vi "Final PID.vi"() -> ()   [LabVIEW 2009, in "Varian Magnet.lvclass"]
uses:
  Varian Magnet.lvclass
  <vilib>/DAQmx/create/channels.llb/DAQmx Create Channel (AO-Voltage-Basic).vi
  <vilib>/DAQmx/configure/timing.llb/DAQmx Timing (Sample Clock).vi
  <vilib>/DAQmx/create/channels.llb/DAQmx Create Channel (AI-Voltage-Basic).vi
  <vilib>/DAQmx/read.llb/DAQmx Read (Analog 1D DBL 1Chan NSamp).vi
  <vilib>/DAQmx/write.llb/DAQmx Write (Analog DBL 1Chan 1Samp).vi
  <vilib>/Analysis/NI_AALBase.lvlib
panel:
  in  "error in":errorcluster
  out "At Field":bool
  in  "stop 2":bool
  in  "Go to Field":bool
  in  "Field Desired (T)":dbl min=0.0 max=1.2 step=0.1
  out "Tesla":dbl(knob) scale=0.0..1.25
  out "Set Field":dbl min=0.0 max=1.25 step=0.001
  out "Magnetic Field":dbl(graph)
  in  "stop":bool
  in  "data":dbl min=-9.0 max=9.0 format="%0.2f"
  # "Big Knob Ranges:\n0  :  0 T\n10:   0T -.3 T \n20:   0T - .55T\n30:   0T - .8 T \n40:   0T - 1.02T \n50: .05T- 1.13T \n60: .25T- >1.13T \n70: .45T- >1.13T"
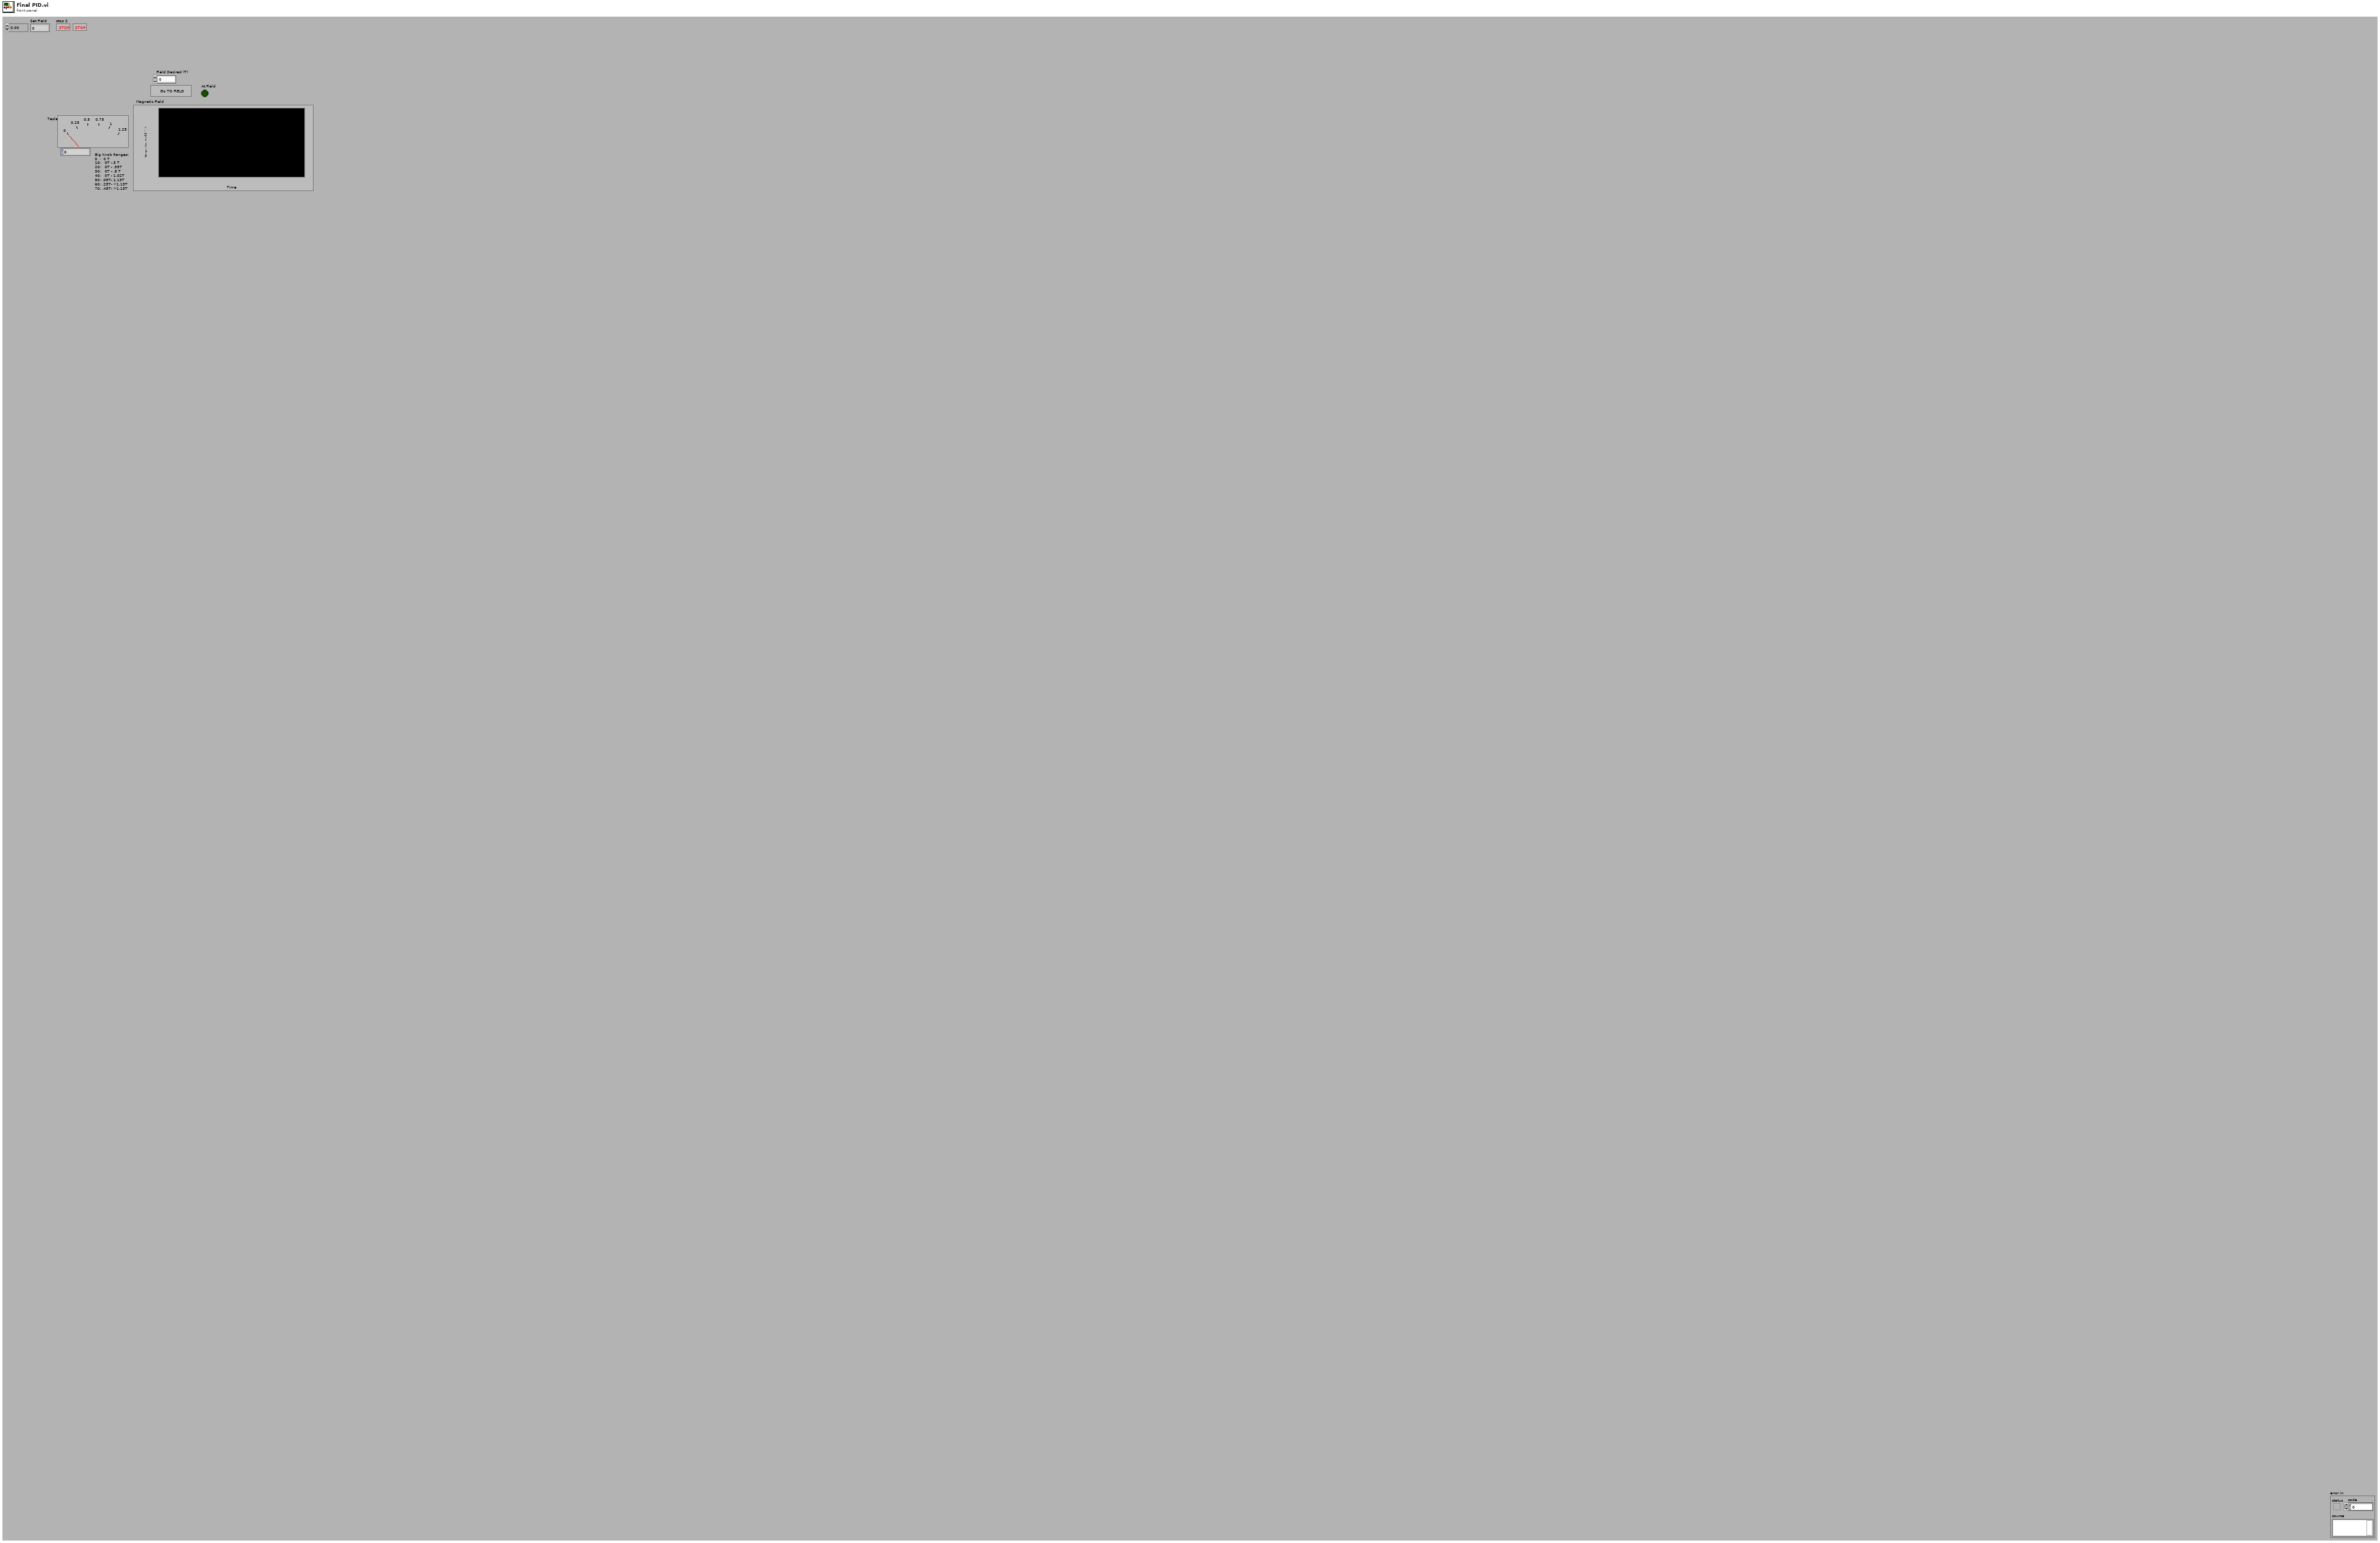
[diagram p1: front panel]
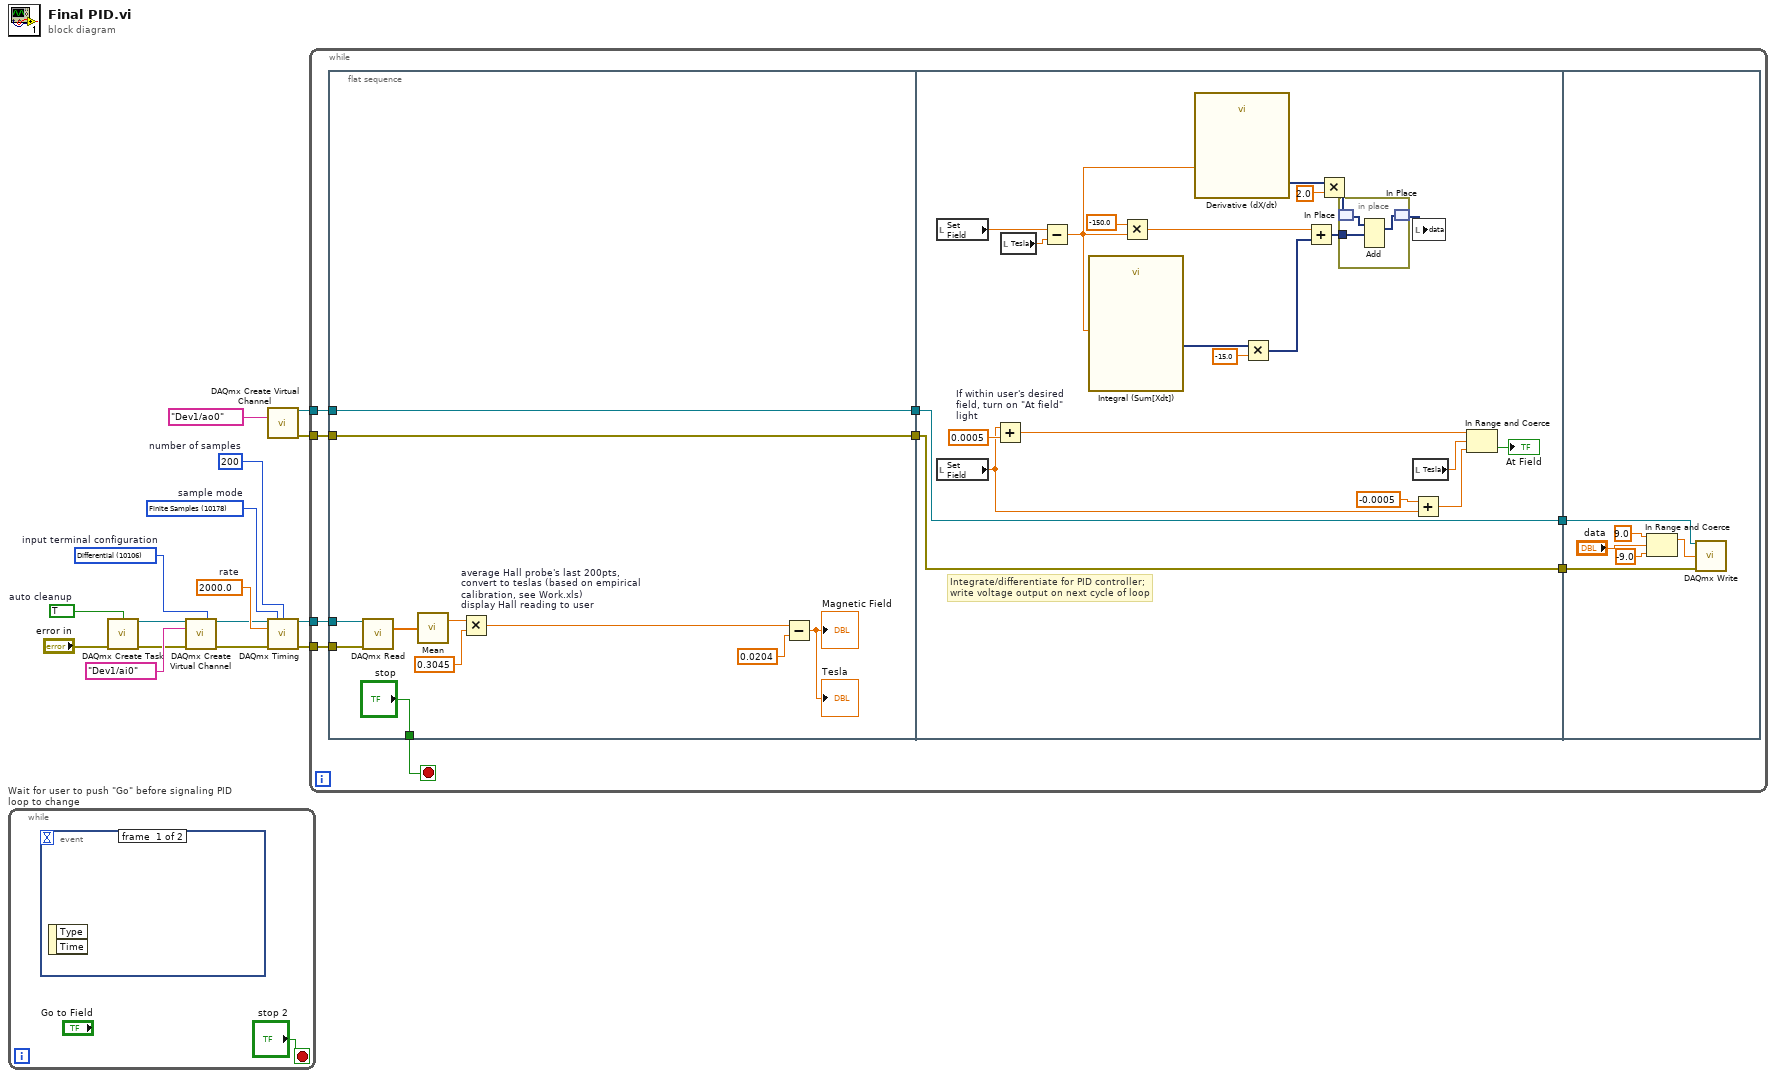
[diagram p0: block diagram]
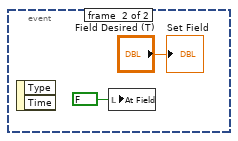
[diagram p2: hidden frame]
diagram:
  w13 = 10178 items=["Finite Samples"=10178, "Continuous Samples"=10123, "Hardware Timed Single Point"=12522]  # sample mode
  w12 = 200  # number of samples
  w11 = 2000.0  # rate
  w4 = 10106 items=["default"=-1, "RSE"=10083, "NRSE"=10078, "Differential"=10106, "Pseudodifferential"=12529]  # input terminal configuration
  w10 = TRUE  # auto cleanup
  n1 = while "Wait for user to push \"Go\" before signaling PID loop to change" {
    stop <- "stop 2" stop-if-true
    n2 = event shown="[1] \"Go to Field\": Value Change" {
      selector: _ -> [_ _]
      dyn-events: _ -> [_ _]
      timeout: _ -> [_ _]
      event #0 {
        n3 = event-data() -> ()  [unwired: 3 out]
      }
      event #1 {
        n4 = event-data() -> ()  [unwired: 3 out]
        n5 = local write "At Field"(FALSE ("At Field")) -> ()
        "Set Field" <- "Field Desired (T)"
      }
    }
  }
  n6 = call <vilib>:"DAQmx Create Task.vi"("auto cleanup"=w10, "error in"="error in") -> ("task out"=w5:refnum<k21>, "error out"=w1:errorcluster)  [unwired: 3 in, 9 out]
  n7 = call-poly <vilib>:"DAQmx Create Virtual Channel.vi"("task in"=w5, "input terminal configuration"=w4, "physical channels"=tag "Dev1/ai0", "error in"=w1) -> ("task out"=w3:refnum<k21>, "error out"=w2:errorcluster)  [unwired: 5 in, 5 out]
  n8 = call-poly <vilib>:"DAQmx Create Virtual Channel.vi"("physical channels"=tag "Dev1/ao0") -> ("task out"=w15:refnum<k21>, "error out"=w16:errorcluster)  [unwired: 8 in, 5 out]
  n9 = call-poly <vilib>:"DAQmx Timing.vi"("task/channels in"=w3, "sample mode"=w13, "samples per channel"=w12, "rate"=w11, "error in"=w2) -> ("task out"=w8:refnum<k21>, "error out"=w7:errorcluster)  [unwired: 2 in, 7 out]
  n10 = while {
    tunnel: w15 -> [w28]
    tunnel: w16 -> [w27]
    tunnel: w8 -> [w21]
    tunnel: w7 -> [w20]
    stop <- w26 stop-if-true
    n11 = flat-sequence {
      tunnel: w28 -> [w32]
      tunnel: w27 -> [w33]
      tunnel: ["stop"] -> w26
      tunnel: [w32] -> w25
      tunnel: [w33] -> w23
      tunnel: w21 -> [w31]
      tunnel: w20 -> [w30]
      tunnel: w25 -> [w41]
      tunnel: [w41] -> w24
      tunnel: w23 -> [w40]
      tunnel: [w40] -> w22
      tunnel: w24 -> [w66]
      tunnel: w22 -> [w65]
      frame #0 {
        n12 = call-poly <vilib>:"DAQmx Read.vi"("task/channels in"=w31, "error in"=w30) -> ("data"=w29:dbl[])  [unwired: 1 in, 12 out]
        n13 = call <vilib>:"Mean.vi"("X"=w29) -> ("mean"=w39:dbl)  [unwired: 1 out]
        n14 = Multiply "average Hall probe's last 200pts,\nconvert to teslas (based on empirical calibration, see Work.xls)\ndisplay Hall reading to user"(x=w39, y=0.3045) -> (x*y=w36:dbl)
        n15 = Subtract(x=w36, y=0.0204 ("x")) -> (x-y=→"Magnetic Field" →"Tesla":dbl)
      }
      frame #1 {
        # "Integrate/differentiate for PID controller;\nwrite voltage output on next cycle of loop"
        n16 = local read "Set Field"() -> (w61:dbl)
        n17 = local read "Set Field"() -> (w44:dbl)
        n18 = Add "If within user's desired field, turn on \"At field\" light"(x=w44, y=0.0005) -> (x+y=w47:dbl)
        n19 = local read "Tesla"() -> (w49:dbl)
        n20 = Subtract(x=w61, y=w49) -> (x-y=w50:dbl)
        n21 = call "Integral (Sum[Xdt])"("Signals"=w50) -> ("Result"=w52:dynamicdata)  [unwired: 1 in, 5 out]
        n22 = Multiply(x=-150.0 ("KP"), y=w50) -> (x*y=w57:dbl)
        n23 = call "Derivative (dX/dt)"("Signals"=w50) -> ("Result"=w51:dynamicdata)  [unwired: 1 in, 5 out]
        n24 = Multiply(x=w52, y=-15.0 ("KI")) -> (x*y=w56:dynamicdata)
        n25 = Add(x=w57, y=w56) -> (x+y=w55:dynamicdata)
        n26 = Multiply(x=w51, y=2.0 ("KD")) -> (x*y=w54:dynamicdata)
        n27 = in-place {
          in-place-border: w55 -> [w64]
          n28 = in-place-match #1(w54) -> (w63:dynamicdata)
          n29 = Add(1:w64, 2:w63) -> (0:w62:dynamicdata)  [unwired: 1 in, 1 out]
          n30 = in-place-match #1(w62) -> (w53:dynamicdata)
        }
        n31 = local write "data"(w53) -> ()
        n32 = local read "Tesla"() -> (w43:dbl)
        n33 = Add(x=-0.0005, y=w44) -> (x+y=w48:dbl)
        n34 = In Range and Coerce(upper limit=w47, x=w43, lower limit=w48) -> (In Range?=→"At Field":bool)  [unwired: 1 out]
      }
      frame #2 {
        n35 = In Range and Coerce(upper limit=9.0 ("y"), x="data", lower limit=-9.0 ("y")) -> (coerced(x)=w70:dbl)  [unwired: 1 out]
        n36 = call-poly <vilib>:"DAQmx Write.vi"("task/channels in"=w66, "data"=w70, "error in"=w65) -> ()  [unwired: 1 in, 12 out]
      }
    }
  }
